vi "UT_Conditionalcheck.vi"() -> ()   [LabVIEW 2014]
uses:
  TableLogger_SQLite_Actor.lvclass
panel:
  out "Label":string[](array[string])
  out "Value":string[](array[string])
  out "error out":errorcluster
  in  "error in (no error)":errorcluster
  out "appended array":variant[](array[variant])
  in  "LV Data":T1={"Numeric Data"=0, "Float Data"=0.0, "String Data"="", "Enum Data"=enum."Enum Item 2", "Array Data 2"=[], "LV Data 2"={"String Data2"="String2", "Array Data"=[2]}}
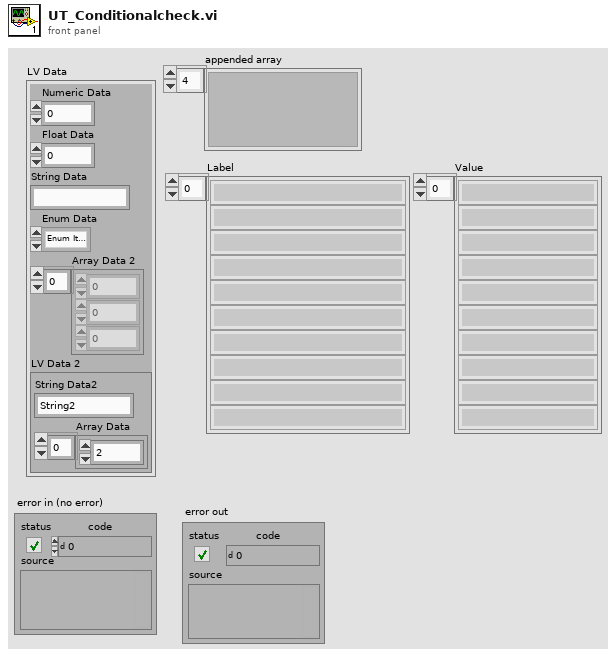
[diagram p1: front panel]
types:
  T1 = cluster{"Numeric Data":i32, "Float Data":dbl, "String Data":string, "Enum Data":enum16{"Enum Item 1", "Enum Item 2"}, "Array Data 2":i32[], "LV Data 2":cluster{"String Data2":string, "Array Data":i32[]}}
  T2 = cluster{"String Data2":string, "Array Data":i32[]}
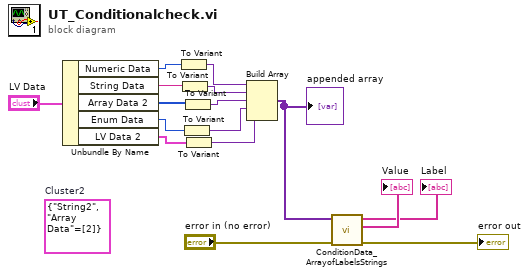
[diagram p0: block diagram]
diagram:
  (unwired) cluster{string, "Array Data":i32[]} {"String2", "Array Data"=[2]}  # Cluster2
  n1 = Unbundle By Name("LV Data") -> ("Numeric Data"=w11:i32, "String Data"=w12:string, "Array Data 2"=w15:i32[], "Enum Data"=w14:enum16{"Enum Item 1", "Enum Item 2"}, "LV Data 2"=w13:T2)
  n2 = To Variant(anything=w11) -> (Variant=w10:variant)
  n3 = To Variant(anything=w12) -> (Variant=w9:variant)
  n4 = To Variant(anything=w14) -> (Variant=w7:variant)
  n5 = To Variant(anything=w15) -> (Variant=w8:variant)
  n6 = To Variant(anything=w13) -> (Variant=w6:variant)
  n7 = Build Array(w10, w9, w8, w7, w6) -> (w5:variant[])
  "appended array" <- w5
  n8 = call "ConditionData_ArrayofLabelsStrings.vi"("error in (no error)"="error in (no error)", "Condition Data"=w5) -> ("error out"=→"error out":errorcluster, "Value"=→"Value":string[], "Label"=→"Label":string[])  [unwired: 7 in]
